vi "SAW peak fit.vi"(11 "in dB":cluster{dbl[], dbl[]}[](graph)) -> ()   [LabVIEW 2020]
uses:
  <userlib>/LevyLab/XY Utilities/subVIs/Subtract XY (single).vi
  <vilib>/gmath/NumericalOptimization/Nonlinear Curve Fit LM.vi
  <vilib>/gmath/NI_Gmath.lvlib
  <userlib>/LevyLab/XY Utilities/xy_utilities.lvlib
panel:
  in  "Reflection?":bool
  in  "Subtract this":cluster{dbl[], dbl[]}[](graph)=[{array[380 elements], array[380 elements]}]
  in  "True for mW":bool
  out "dip data":cluster{i32[], dbl[]}[](graph)
  out "Qfac":cluster{i32[], dbl[]}[](graph)
  out "Bandwidth":cluster{i32[], dbl[]}[](graph)
  out "S dip from fit":cluster{i32[], dbl[]}[](graph)
  out "Fits":cluster{dbl[], "f(X,a)":dbl[]}[](graph)
  out "fc from fit":cluster{i32[], dbl[]}[](graph)
  out "number of function calls":i32=531
  out "residue":dbl=0.9474933142146692
  out "Data and fit":cluster{dbl[], "f(X,a)":dbl[]}[](graph)
  out "Parameter Guess":dbl[](array[numeric])=[320633931.25, 13124956.25, 7.446533203125, 0.0] caption="pos\nwidth\namplitude*\noffset" format="%.4e"
  out "best fit parameters":dbl[](array[numeric])=[321940516.2554543, 33489259.319360655, 7.954631946080219, -0.514086965480449] caption="pos\nwidth\nheight\noffset" format="%.4e"
  out "After subtract 300K":cluster{dbl[], dbl[]}[](graph)
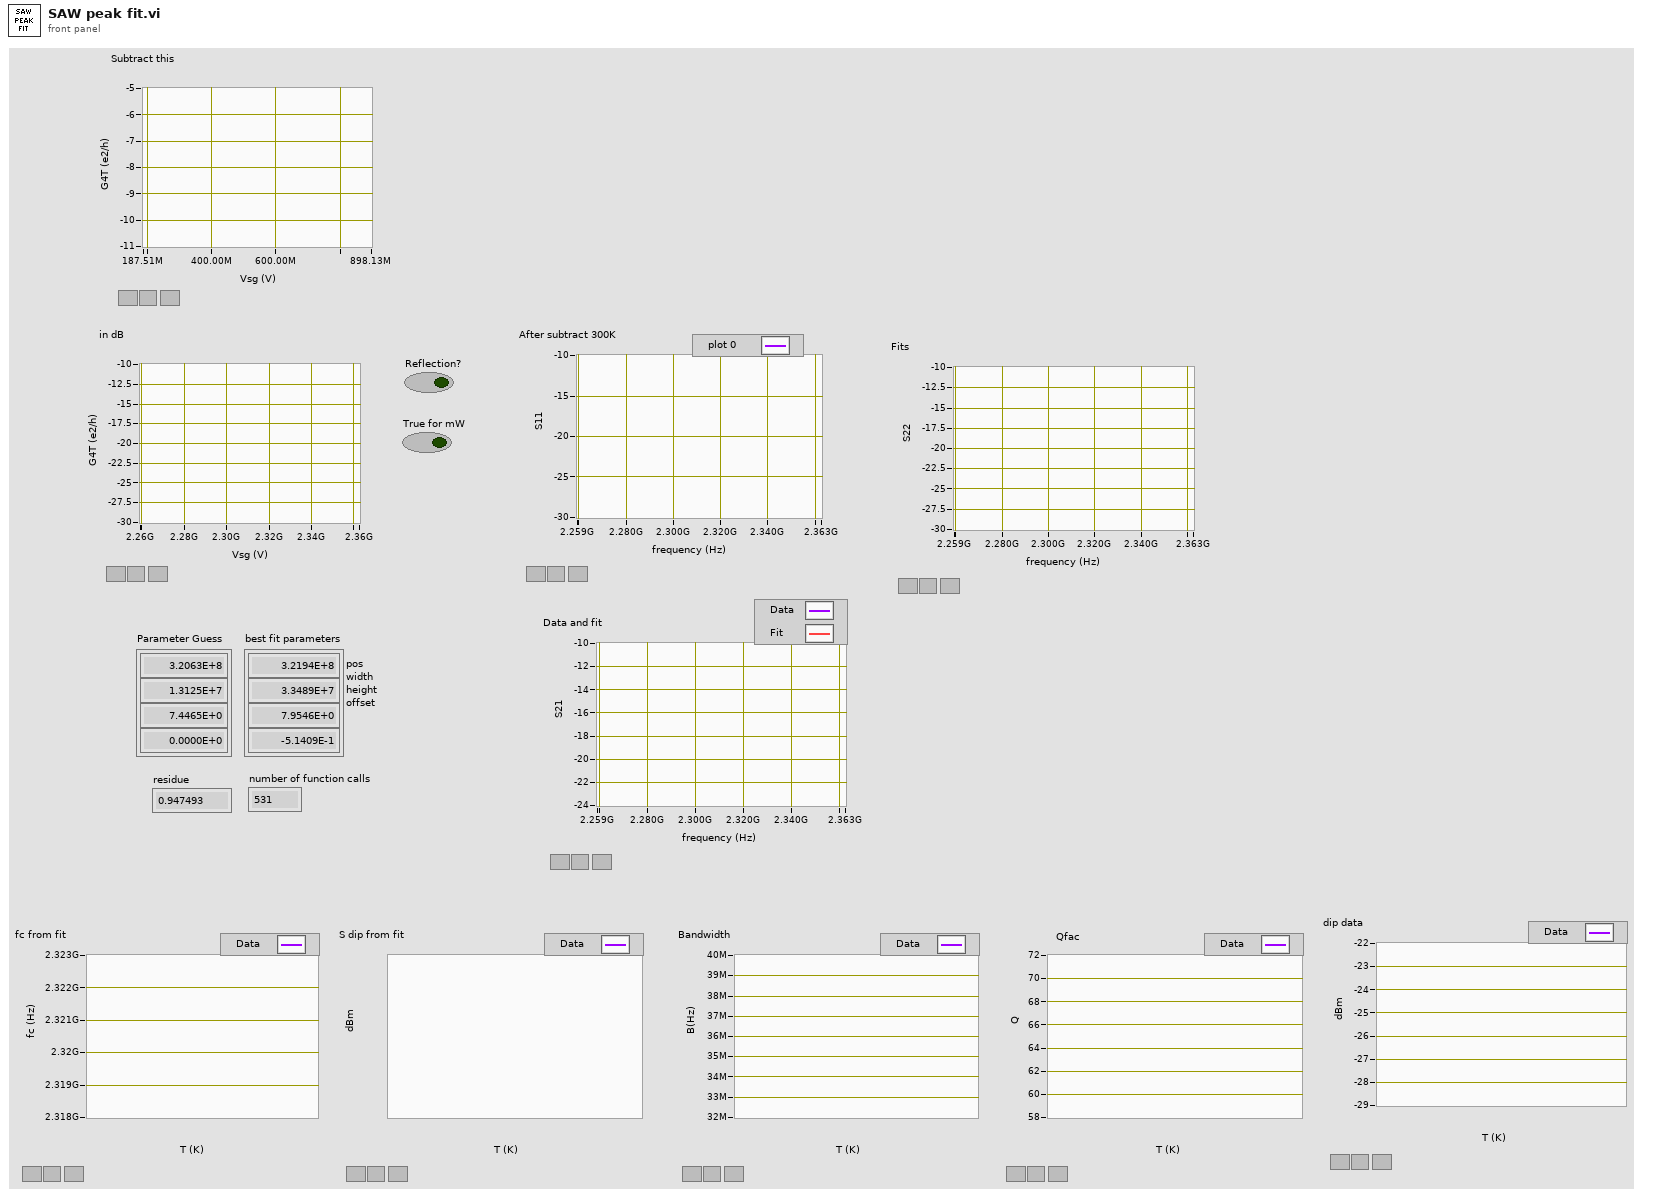
[diagram p1: front panel]
types:
  T1 = cluster{"X-array":dbl[], "best nonlinear fit":dbl[]}
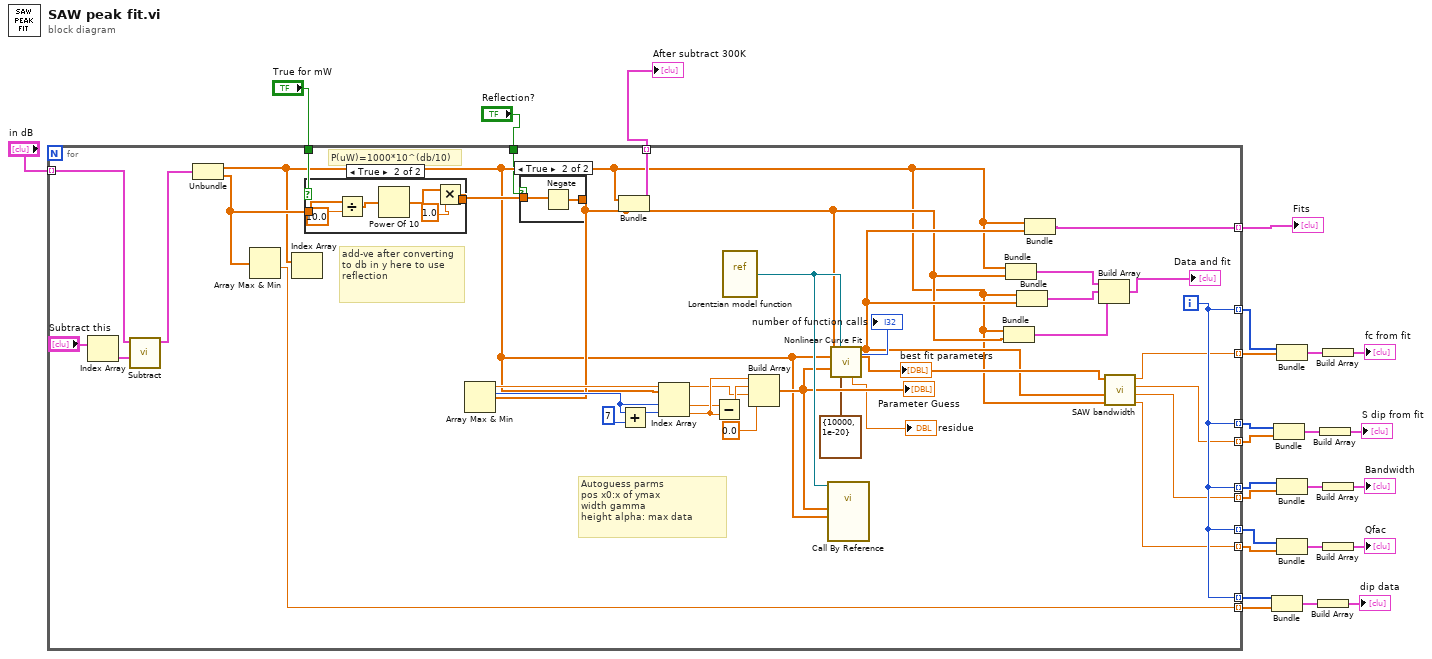
[diagram p0: block diagram]
diagram:
  n1 = for {
    tunnel: "in dB" -> [w29] mode=indexing
    tunnel: [w62] -> w24 mode=indexing
    tunnel: [w38] -> w23 mode=indexing
    tunnel: [w43] -> w22 mode=indexing
    tunnel: [w46] -> w20 mode=indexing
    tunnel: [w43] -> w17 mode=indexing
    tunnel: [w43] -> w16 mode=indexing
    tunnel: [w37] -> w15 mode=indexing
    tunnel: [w35] -> w10 mode=indexing
    tunnel: [w43] -> w14 mode=indexing
    tunnel: [w43] -> w13 mode=indexing
    tunnel: [w27] -> w11 mode=indexing
    tunnel: [w36] -> w9 mode=indexing
    tunnel: "True for mW" -> [w34]
    tunnel: "Reflection?" -> [w26]
    i -> [w43]
    # "add-ve after converting to db in y here to use reflection"
    # "Autoguess parms\npos x0:x of ymax\nwidth gamma\nheight alpha: max data"
    # "P(uW)=1000*10^(db/10)"
    n2 = Index Array(array="Subtract this") -> (element=w30:cluster{dbl[], dbl[]})  [unwired: 1 in]
    n3 = call-poly <userlib>:"Subtract.vi"("y"=w30, "XY-data"=w29) -> ("XY-data out"=w28:cluster{"X-array":dbl[], "Y-array":dbl[]})  [unwired: 8 in, 1 out]
    n4 = Unbundle(w28) -> ("X-array"=w32:dbl[], "Y-array"=w33:dbl[])
    n5 = Array Max & Min(array=w33) -> (min value=w27:dbl)  [unwired: 3 out]
    n6 = Index Array(array=w32) -> ()  [unwired: 1 in, 1 out]
    n7 = case shown="True" w34 {
      tunnel: [w66 w68] -> w45
      tunnel: w33 -> [w66 w67]
      frame False {
      }
      frame True {
        n8 = Divide(x=w67, y=10.0) -> (x/y=w71:dbl[])
        n9 = Power Of 10(x=w71) -> (10^x=w69:dbl[])
        n10 = Multiply(x=w69, y=1.0) -> (x*y=w68:dbl[])
      }
    }
    n11 = case shown="True" w26 {
      tunnel: w45 -> [w63 w65]
      tunnel: [w63 w64] -> w39
      frame False {
      }
      frame True {
        n12 = Negate(x=w65) -> (-x=w64:dbl[])
      }
    }
    n13 = Array Max & Min(array=w39) -> (max value=w44:dbl, max index (indices)=w61:i32)  [unwired: 2 out]
    n14 = Bundle("X-array"=w32, "Y-array"=w39) -> (w62:cluster{"X-array":dbl[], "Y-array":dbl[]})  [unwired: 1 in]
    n15 = Add(x=w61, y=7) -> (x+y=w60:i32)
    n16 = Index Array(array=w32, index #1=w61, index #2=w60) -> (element #1=w58:dbl, element #2=w57:dbl)
    n17 = Subtract(x=w57, y=w58) -> (x-y=w56:dbl)
    n18 = vi-ref "Lorentzian model function.vi"() -> (w55:refnum<vi>)
    n19 = Build Array(w58, w56, w44, 0.0 ("element")) -> (w54:dbl[])
    "Parameter Guess" <- w54
    n20 = call-by-ref "?"(reference=w55, "X"=w32, "a"=w54) -> ()  [unwired: 3 in, 5 out]
    n21 = call-poly <vilib>:"Nonlinear Curve Fit.vi"("Y"=w39, "f(x,a)"=w55, "X"=w32, "initial parameters"=w54, "termination"=cluster{"max iteration":i32, "tolerance":dbl} {"max iteration"=10000, "tolerance"=1e-20}) -> ("number of function calls"=→"number of function calls":i32, "best nonlinear fit"=w40:dbl[], "best fit parameters"=w41:dbl[], "residue"=→"residue":dbl)  [unwired: 5 in, 2 out]
    "best fit parameters" <- w41
    n22 = Bundle("X-array"=w32, "Y-array"=w39) -> (w52:cluster{"X-array":dbl[], "Y-array":dbl[]})  [unwired: 1 in]
    n23 = Bundle("X-array"=w32, "Y-array"=w39) -> (w53:cluster{"X-array":dbl[], "Y-array":dbl[]})  [unwired: 1 in]
    n24 = Bundle("X-array"=w32, "best nonlinear fit"=w40) -> (w47:T1)  [unwired: 1 in]
    n25 = Bundle("X-array"=w32, "best nonlinear fit"=w40) -> (w46:T1)  [unwired: 1 in]
    n26 = Build Array(w53, w47, w52) -> (→"Data and fit":cluster{"X-array":dbl[], "Y-array":dbl[]}[])
    n27 = call "SAW bandwidth.vi"("x array"=w32, "best fit y"=w40, "best fit parms"=w41) -> ("Q factor"=w35:dbl, "Bandwidth"=w36:dbl, "S11 dip"=w37:dbl, "fc from fit"=w38:dbl)  [unwired: 5 in]
  }
  "After subtract 300K" <- w24
  "Fits" <- w20
  n28 = Bundle(w13, w11) -> (w12:cluster{i32[], dbl[]})  [unwired: 1 in]
  n29 = Bundle(w17, w15) -> (w19:cluster{i32[], dbl[]})  [unwired: 1 in]
  n30 = Bundle(w22, w23) -> (w21:cluster{i32[], dbl[]})  [unwired: 1 in]
  n31 = Bundle(w16, w9) -> (w18:cluster{i32[], dbl[]})  [unwired: 1 in]
  n32 = Bundle(w14, w10) -> (w7:cluster{i32[], dbl[]})  [unwired: 1 in]
  n33 = Build Array(w12) -> (→"dip data":cluster{i32[], dbl[]}[])
  n34 = Build Array(w19) -> (→"S dip from fit":cluster{i32[], dbl[]}[])
  n35 = Build Array(w21) -> (→"fc from fit":cluster{i32[], dbl[]}[])
  n36 = Build Array(w18) -> (→"Bandwidth":cluster{i32[], dbl[]}[])
  n37 = Build Array(w7) -> (→"Qfac":cluster{i32[], dbl[]}[])
